vi "E2-2.vi"() -> ()   [LabVIEW 2011]
panel:
  out "A/B":dbl
  out "A*B":dbl
  out "A-B":dbl
  out "A+B":dbl
  in  "B":dbl
  in  "A":dbl
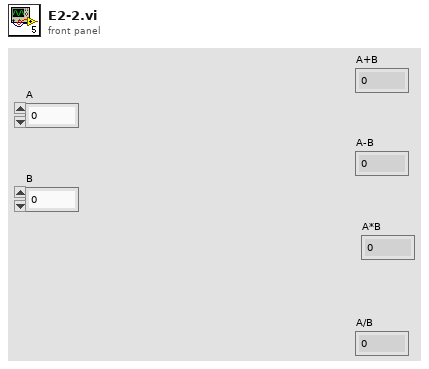
[diagram p1: front panel]
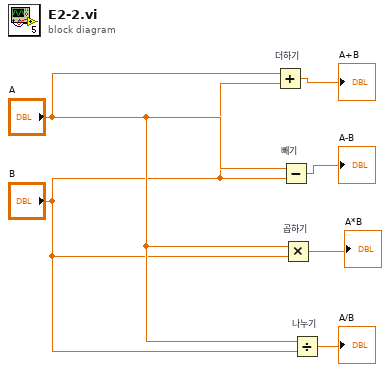
[diagram p0: block diagram]
diagram:
  n1 = Add "더하기"(x="A", y="B") -> (x+y=→"A+B":dbl)
  n2 = Subtract "빼기"(x="A", y="B") -> (x-y=→"A-B":dbl)
  n3 = Multiply "곱하기"(x="A", y="B") -> (x*y=→"A*B":dbl)
  n4 = Divide "나누기"(x="A", y="B") -> (x/y=→"A/B":dbl)
